vi "WD_Set_L_NULL.vi"(8 "error in (no error)":errorcluster, 10 "Barcode L":string, 11 "DBlink":string="Driver={ODBC Driver 17 for SQL Server};Server=localhost\\SQLEXPRESS;Database=ZDX201;UID=labview;PWD=Dsa@54137926") -> (0 "error out":errorcluster, 2 "Workplace: assemble":cluster{"條碼A":string, "條碼B":string}[](array[cluster]))   [LabVIEW 2019]
uses:
  <vilib>/addons/database/Connection.llb/DB Tools Open Connec (String).vi
  <vilib>/addons/database/Connection.llb/Conn Execute.vi
  <vilib>/addons/database/Recordset.llb/Rec Fetch Recordset Data (R).vi
  <vilib>/addons/database/Recordset.llb/Rec Destroy - Connection.vi
  <vilib>/addons/database/_DB Variant To Data/Database Variant To Data.xnode
  <vilib>/addons/database/NI_Database_API.lvlib
panel:
  out "查詢結果":string="Update [workplace_data] \nset  \n[barcode A] = NULL       \n  ,[barcode B] = NULL\n"
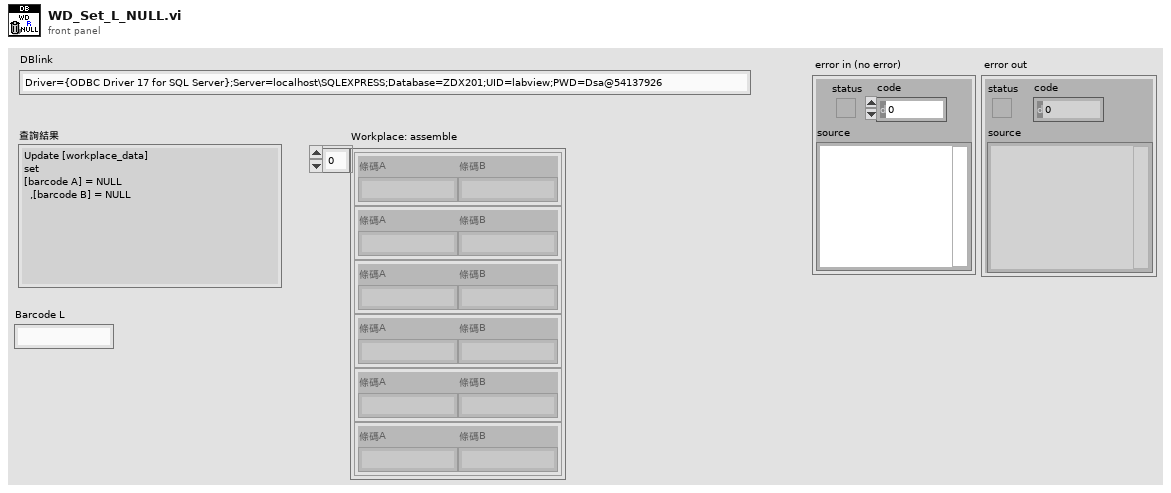
[diagram p1: front panel]
types:
  T1 = typedef "NI_Database_API.lvlib/Conn ObjectReference.ctl" = refnum<k1>
  T2 = typedef "NI_Database_API.lvlib/Rec ObjectReference.ctl" = refnum<k1>
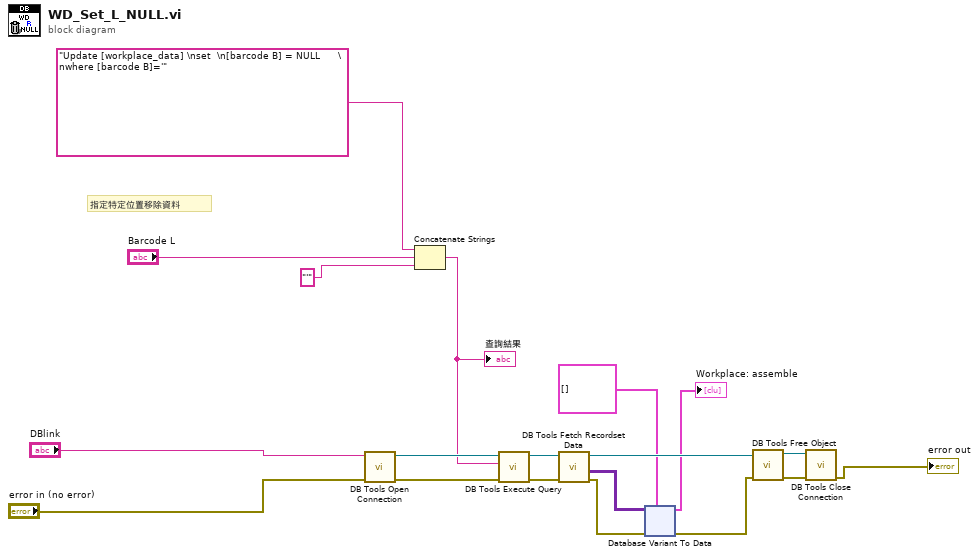
[diagram p0: block diagram]
diagram:
  # "指定特定位置移除資料"
  n1 = call-poly <vilib>:"DB Tools Open Connection.vi"("error in (no error)"="error in (no error)", "connection information"="DBlink") -> ("error out"=w19:errorcluster, "connection reference"=w18:T1)  [unwired: 6 in]
  n2 = Concatenate Strings("Update [workplace_data] \nset  \n[barcode B] = NULL      \nwhere [barcode B]='", "Barcode L", "'") -> (w3:string)
  "查詢結果" <- w3
  n3 = call-poly <vilib>:"DB Tools Execute Query.vi"("error in (no error)"=w19, "SQL query"=w3, "connection reference"=w18) -> ("error out"=w16:errorcluster, "recordset reference"=w17:T2)  [unwired: 5 in]
  n4 = call-poly <vilib>:"DB Tools Fetch Recordset Data.vi"("error in (no error)"=w16, "recordset reference"=w17) -> ("error out"=w11:errorcluster, "recordset data"=w10:variant[][], "recordset reference out"=w12:T2)  [unwired: 3 in]
  n5 = xnode "Database Variant To Data"("database variant"=w10, "error in (no error)"=w11, "type"=cluster{"條碼A":string, "條碼B":string}[] [] ("Workplace: assemble")) -> ("data"=→"Workplace: assemble":cluster{"條碼A":string, "條碼B":string}[], "error out"=w13:errorcluster)
  n6 = call-poly <vilib>:"DB Tools Free Object.vi"("error in (no error)"=w13, "recordset reference"=w12) -> ("error out"=w14:errorcluster, "connection reference"=w15:T1)  [unwired: 8 in]
  n7 = call <vilib>:"DB Tools Close Connection.vi"("error in (no error)"=w14, "connection reference"=w15) -> ("error out"=→"error out":errorcluster)  [unwired: 5 in]
